vi "solar_misc Image Overlay.vi"(10 "Overlay":T1, 11 "Image":T1) -> (2 "new picture":picture, 3 "Image with Overlay":T1)   [LabVIEW 2018]
doc: "This VI adds an overlay image to the bottom right of the original image."
uses:
  <vilib>/picture/picture.llb/imagedata.ctl
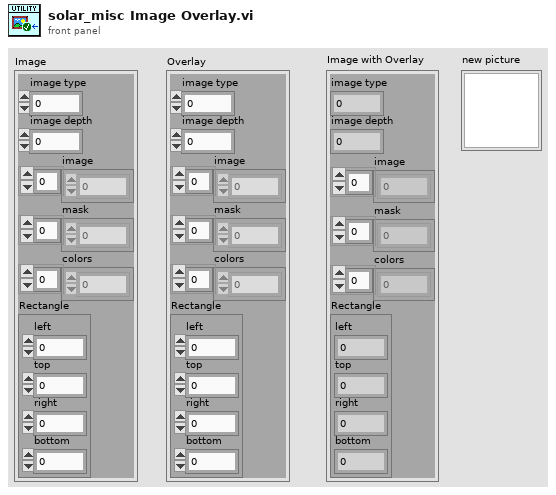
[diagram p1: front panel]
types:
  T1 = typedef "imagedata.ctl" = cluster{"image type":i32, "image depth":i32, "image":u8[], "mask":u8[], "colors":u32[], "Rectangle":cluster{"left":i16, "top":i16, "right":i16, "bottom":i16}}
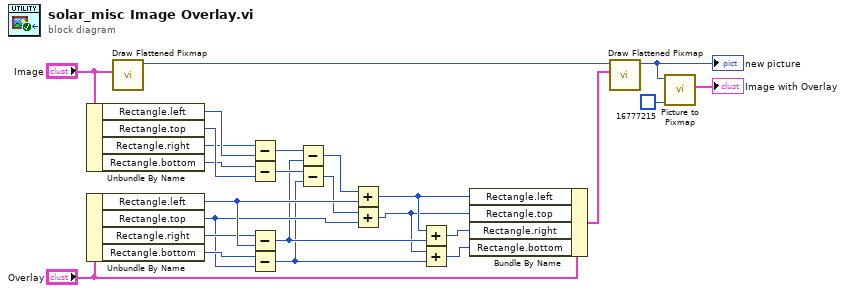
[diagram p0: block diagram]
diagram:
  n1 = Unbundle By Name("Image") -> ("Rectangle.left"=w23:i16, "Rectangle.top"=w22:i16, "Rectangle.right"=w20:i16, "Rectangle.bottom"=w21:i16)
  n2 = Unbundle By Name("Overlay") -> ("Rectangle.left"=w16:i16, "Rectangle.top"=w11:i16, "Rectangle.right"=w14:i16, "Rectangle.bottom"=w24:i16)
  n3 = call <vilib>:"Draw Flattened Pixmap.vi"("image data"="Image") -> ("new picture"=w25:picture)  [unwired: 8 in]
  n4 = Subtract(x=w20, y=w23) -> (x-y=w18:i16)
  n5 = Subtract(x=w21, y=w22) -> (x-y=w17:i16)
  n6 = Subtract(x=w14, y=w16) -> (x-y=w9:i16)
  n7 = Subtract(x=w24, y=w11) -> (x-y=w6:i16)
  n8 = Subtract(x=w18, y=w9) -> (x-y=w15:i16)
  n9 = Subtract(x=w17, y=w6) -> (x-y=w10:i16)
  n10 = Add(x=w15, y=w16) -> (x+y=w8:i16)
  n11 = Add(x=w10, y=w11) -> (x+y=w7:i16)
  n12 = Add(x=w8, y=w9) -> (x+y=w12:i16)
  n13 = Add(x=w7, y=w6) -> (x+y=w5:i16)
  n14 = Bundle By Name(cluster="Overlay", "Rectangle.left"=w8, "Rectangle.top"=w7, "Rectangle.right"=w12, "Rectangle.bottom"=w5) -> (w4:T1)
  n15 = call <vilib>:"Draw Flattened Pixmap.vi"("image data"=w4, "picture"=w25) -> ("new picture"=w3:picture)  [unwired: 7 in]
  "new picture" <- w3
  n16 = call <vilib>:"Picture to Pixmap.vi"("Background Color"=u32 16777215, "picture"=w3) -> ("image data"=→"Image with Overlay":T1)  [unwired: 8 in, 1 out]
